vi "read_DB_small.vi"(8 "error in (no error)":errorcluster, 10 "Dust event ID":i64) -> (0 "error out":errorcluster, 2 "Cluster":T1 {"File Location" items=["Unknown"=-5, "IDL Processing"=-4, "Writing from Queue"=-3, "Labview Files"=-2, "Retry Labview files"=-1, "Local Cache "=0, "Storage"=1]})   [LabVIEW 2013]
uses:
  Post_Dust_Event_small.ctl
  Private/Controls/File_location.ctl
  <vilib>/addons/database/Connection.llb/Conn Execute.vi
  <vilib>/addons/database/Recordset.llb/Rec Fetch Recordset Data (R).vi
  <vilib>/addons/database/Recordset.llb/Rec Destroy - Connection.vi
  <vilib>/addons/database/_DB Variant To Data/Database Variant To Data.xnode
  <vilib>/addons/database/NI_Database_API.lvlib
panel:
  # "Dust Event Small"
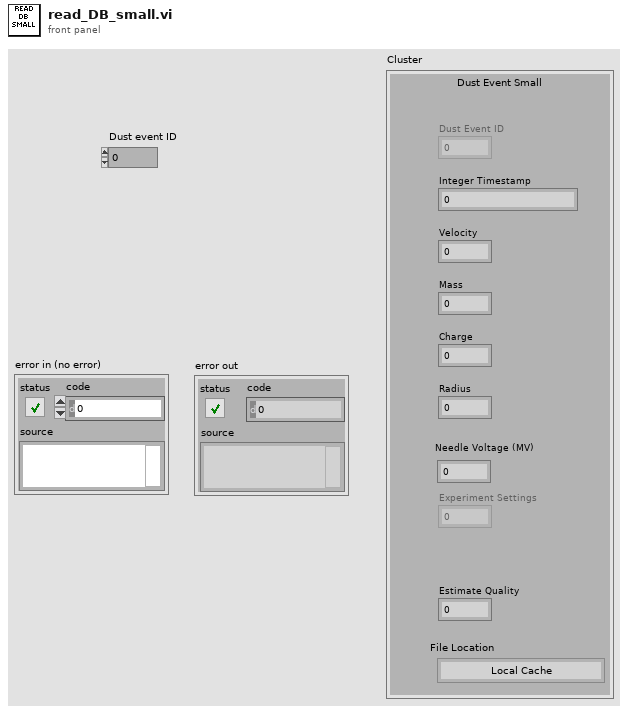
[diagram p1: front panel]
types:
  T1 = typedef "Post_Dust_Event_small.ctl" = cluster{"Dust Event ID":i64, "Integer Timestamp":i64, "Velocity":sgl, "Mass":sgl, "Charge":sgl, "Radius":sgl, "Needle Voltage (MV)":dbl, "Experiment Settings":dbl, "Estimate Quality":sgl, "File Location":T2, "id_dust_info":dbl}
  T2 = typedef "File_location.ctl" = i8
  T3 = typedef "NI_Database_API.lvlib/Conn ObjectReference.ctl" = refnum<k1>
  T4 = typedef "NI_Database_API.lvlib/Rec ObjectReference.ctl" = refnum<k1>
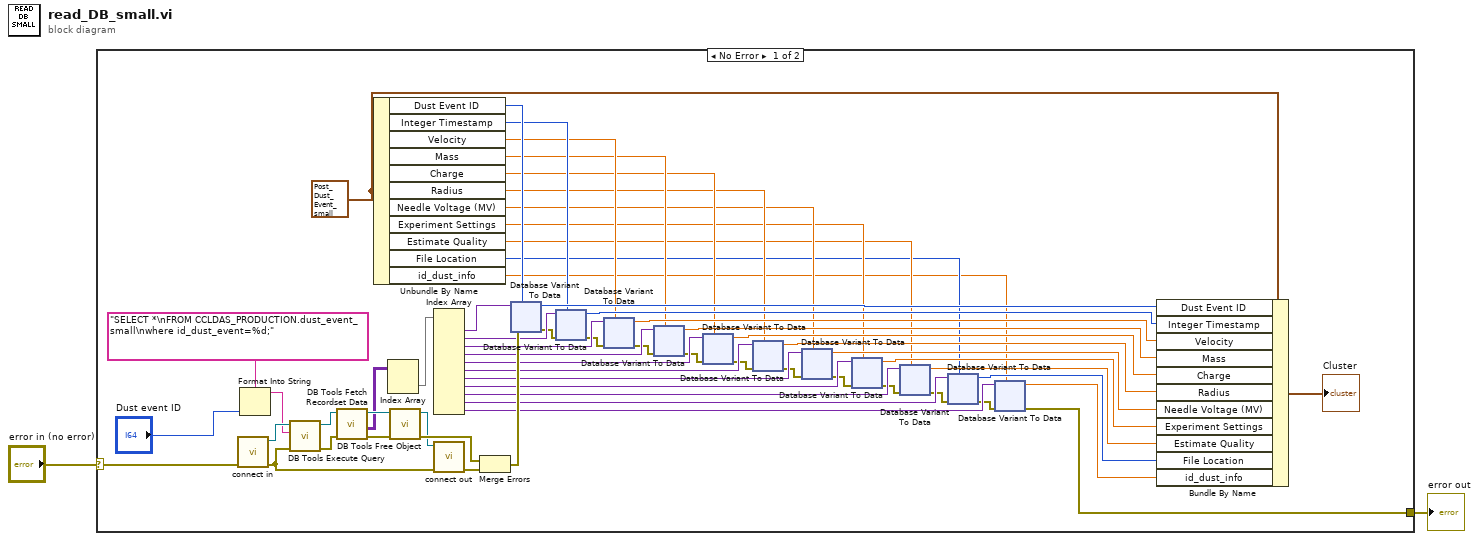
[diagram p0: block diagram]
diagram:
  n1 = case shown="No Error" "error in (no error)" {
    selector: "error in (no error)" -> [w64 w417]
    tunnel: [w4 w417] -> w2
    frame No Error {
      w27 = T1 {"Dust Event ID"=0, "Integer Timestamp"=0, "Velocity"=0.0, "Mass"=0.0, "Charge"=0.0, "Radius"=0.0, "Needle Voltage (MV)"=0.0, "Experiment Settings"=0.0, "Estimate Quality"=0.0, "File Location"=0, "id_dust_info"=0.0} ("Cluster")
      n2 = call "connect in.vi"("error in (no error)"=w64) -> ("error out"=w61:errorcluster, "Database Connection"=w60:T3)  [unwired: 6 in, 1 out]
      n3 = Format Into String(format string="SELECT *\nFROM CCLDAS_PRODUCTION.dust_event_small\nwhere id_dust_event=%d;", "Dust event ID") -> (resulting string=w53:string)  [unwired: 2 in, 1 out]
      n4 = call-poly <vilib>:"DB Tools Execute Query.vi"("error in (no error)"=w61, "SQL query"=w53, "connection reference"=w60) -> ("error out"=w59:errorcluster, "recordset reference"=w58:T4)  [unwired: 5 in]
      n5 = call-poly <vilib>:"DB Tools Fetch Recordset Data.vi"("error in (no error)"=w59, "recordset reference"=w58) -> ("error out"=w57:errorcluster, "recordset data"=w52:variant[][], "recordset reference out"=w56:T4)  [unwired: 3 in]
      n6 = Unbundle By Name(w27) -> ("Dust Event ID"=w15:i64, "Integer Timestamp"=w14:i64, "Velocity"=w13:sgl, "Mass"=w12:sgl, "Charge"=w11:sgl, "Radius"=w10:sgl, "Needle Voltage (MV)"=w9:dbl, "Experiment Settings"=w8:dbl, "Estimate Quality"=w7:sgl, "File Location"=w6:T2, "id_dust_info"=w5:dbl)
      n7 = Index Array(array=w52) -> (element=w50:variant[])  [unwired: 2 in]
      n8 = call-poly <vilib>:"DB Tools Free Object.vi"("error in (no error)"=w57, "recordset reference"=w56) -> ("error out"=w62:errorcluster, "connection reference"=w51:T3)  [unwired: 8 in]
      n9 = Index Array(array=w50) -> (element #1=w49:variant, element #2=w47:variant, element #3=w45:variant, element #4=w43:variant, element #5=w41:variant, element #6=w39:variant, element #7=w37:variant, element #8=w35:variant, element #9=w33:variant, element #10=w31:variant, element #11=w29:variant)  [unwired: 11 in]
      n10 = call "connect out.vi"("error in (no error)"=w61, "connection reference"=w51) -> ("error out"=w63:errorcluster)  [unwired: 9 in]
      n11 = Merge Errors(w62, w63) -> (w48:errorcluster)
      n12 = xnode "Database Variant To Data"("database variant"=w49, "error in (no error)"=w48, "type"=w15) -> ("data"=w26:i64, "error out"=w46:errorcluster)
      n13 = xnode "Database Variant To Data"("database variant"=w47, "error in (no error)"=w46, "type"=w14) -> ("data"=w25:i64, "error out"=w44:errorcluster)
      n14 = xnode "Database Variant To Data"("database variant"=w45, "error in (no error)"=w44, "type"=w13) -> ("data"=w24:sgl, "error out"=w42:errorcluster)
      n15 = xnode "Database Variant To Data"("database variant"=w43, "error in (no error)"=w42, "type"=w12) -> ("data"=w23:sgl, "error out"=w40:errorcluster)
      n16 = xnode "Database Variant To Data"("database variant"=w41, "error in (no error)"=w40, "type"=w11) -> ("data"=w22:sgl, "error out"=w38:errorcluster)
      n17 = xnode "Database Variant To Data"("database variant"=w39, "error in (no error)"=w38, "type"=w10) -> ("data"=w21:sgl, "error out"=w36:errorcluster)
      n18 = xnode "Database Variant To Data"("database variant"=w37, "error in (no error)"=w36, "type"=w9) -> ("data"=w20:dbl, "error out"=w34:errorcluster)
      n19 = xnode "Database Variant To Data"("database variant"=w35, "error in (no error)"=w34, "type"=w8) -> ("data"=w19:dbl, "error out"=w32:errorcluster)
      n20 = xnode "Database Variant To Data"("database variant"=w33, "error in (no error)"=w32, "type"=w7) -> ("data"=w18:sgl, "error out"=w30:errorcluster)
      n21 = xnode "Database Variant To Data"("database variant"=w31, "error in (no error)"=w30, "type"=w6) -> ("data"=w16:T2, "error out"=w28:errorcluster)
      n22 = xnode "Database Variant To Data"("database variant"=w29, "error in (no error)"=w28, "type"=w5) -> ("data"=w17:dbl, "error out"=w4:errorcluster)
      n23 = Bundle By Name(cluster=w27, "Dust Event ID"=w26, "Integer Timestamp"=w25, "Velocity"=w24, "Mass"=w23, "Charge"=w22, "Radius"=w21, "Needle Voltage (MV)"=w20, "Experiment Settings"=w19, "Estimate Quality"=w18, "File Location"=w16, "id_dust_info"=w17) -> (→"Cluster":T1)
    }
    frame Error {
    }
  }
  "error out" <- w2
